vi "Sensor_Read_Val.vi"(10 "Ele_At_Pos":bool, 11 "Ref_Num":T23) -> (3 "Sensor_Val":T24)   [LabVIEW 2014]
uses:
  <vilib>/Rock Robotics/WPI/Joystick/WPI_JoystickDevRef.ctl
  <vilib>/Rock Robotics/WPI/Joystick/WPI_JoystickDeviceEnum.ctl
  <vilib>/Rock Robotics/WPI/RobotDrive/WPI_RobotDriveDevRef.ctl
  <vilib>/Rock Robotics/WPI/MotorControl/WPI_MotorControlDeviceRef.ctl
  <vilib>/Rock Robotics/WPI/MotorControl/WPI_MotorControlType.ctl
  <vilib>/Rock Robotics/SystemInterfaces/Typedef/FPGA_TypedefDigitalModule.ctl
  <vilib>/Rock Robotics/SystemInterfaces/DIO/FPGA_DIOPWMChannel.ctl
  <vilib>/Rock Robotics/WPI/PWM/WPI_PWMDeadband.ctl
  <vilib>/Rock Robotics/WPI/CAN/Jaguar/SubVIs/WPI_CANJaguar_ControlMode.ctl
  <vilib>/Rock Robotics/WPI/CAN/TalonSRX/WPI_CANTalonSRX_APIControlMode.ctl
  <vilib>/Rock Robotics/WPI/PWM/WPI_PWMTransform_ConPane.ctl
  <vilib>/Rock Robotics/WPI/Encoder/WPI_EncoderDevRef.ctl
  <vilib>/Rock Robotics/SystemInterfaces/Encoder/FPGA_EncoderIdx.ctl
  <vilib>/Rock Robotics/SystemInterfaces/Counter/FPGA_CounterCtrSystemIndex.ctl
  <vilib>/Rock Robotics/WPI/Encoder/WPI_EncoderType.ctl
  <vilib>/Rock Robotics/WPI/AnalogChannel/WPI_AnalogChannelDevRef.ctl
  <vilib>/Rock Robotics/SystemInterfaces/Typedef/FPGA_TypedefAnalogModule.ctl
  <vilib>/Rock Robotics/SystemInterfaces/AI/FPGA_AIChannel.ctl
  <vilib>/Rock Robotics/WPI/Gyro/WPI_GyroDevRef.ctl
  AdaIMU roboRIO/IMUDevRef.ctl
  <vilib>/Rock Robotics/SystemInterfaces/i2clib/i2c_bus.ctl
panel:
  in  "Reset Zero Position 2":bool
  in  "Detect_Tote_Thresh_Hold":dbl
  in  "Yoyo_Scale_to_Inch":dbl
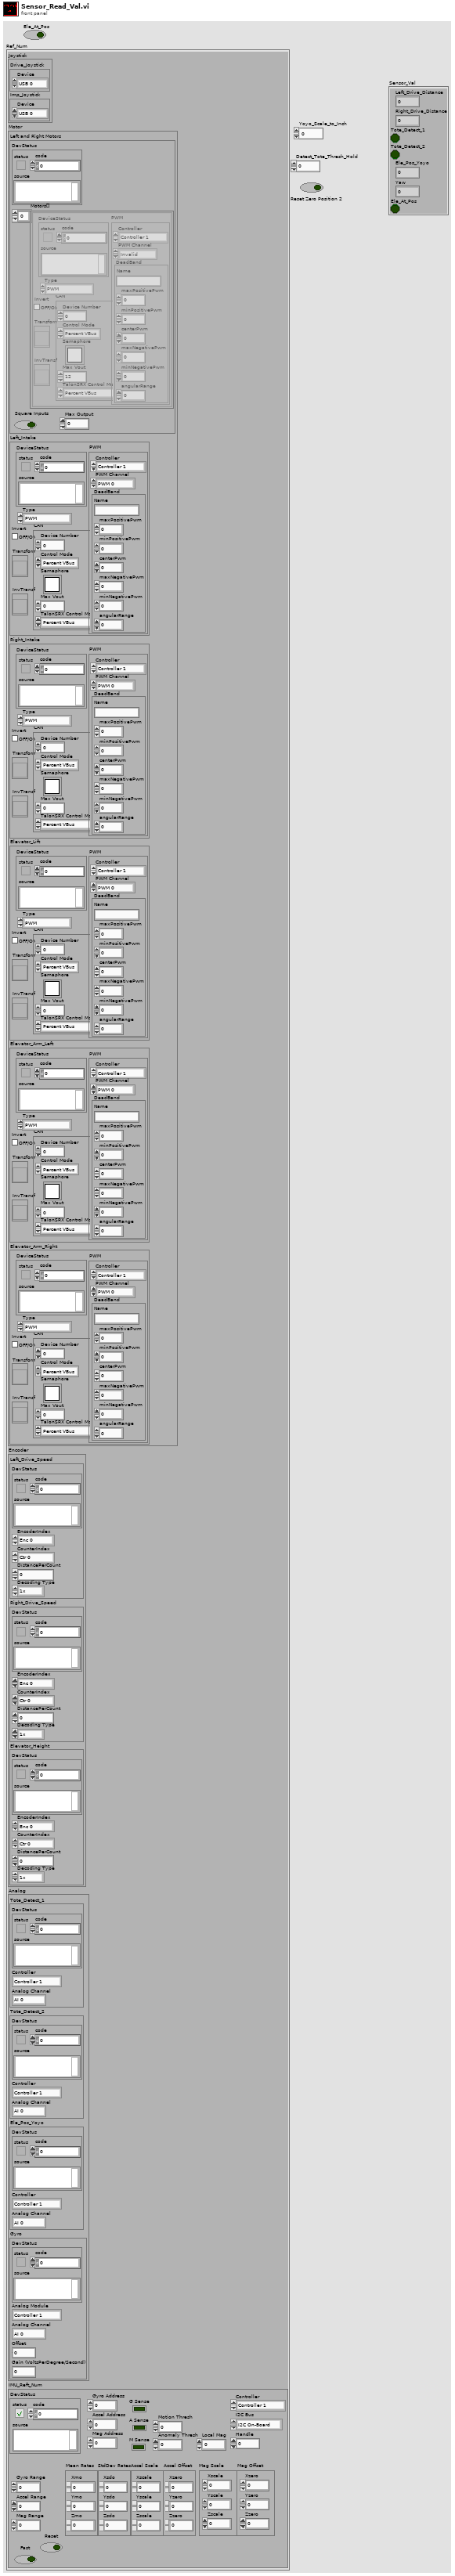
[diagram p1: front panel]
types:
  T1 = typedef "WPI_JoystickDevRef.ctl" = cluster{"Device":T2}
  T2 = typedef "WPI_JoystickDeviceEnum.ctl" = enum16{"USB 0", "USB 1", "USB 2", "USB 3", "USB 4", "USB 5"}
  T3 = typedef "WPI_RobotDriveDevRef.ctl" = cluster{"DevStatus":errorcluster, "Motors[]":T4[], "Square Inputs":bool, "Max Output":dbl}
  T4 = typedef "WPI_MotorControlDeviceRef.ctl" = cluster{"DeviceStatus":errorcluster, "Type":T5, "PWM":cluster{"Controller":T6, "PWM Channel":T7, "DeadBand":T8}, "CAN":cluster{"Device Number":u8, "Control Mode":T9, "Semaphore":T10, "Max Vout":dbl, "TalonSRX Control Mode":T11}, "Invert":bool, "TransformRef":T12, "InvTransformRef":T12}
  T5 = typedef "WPI_MotorControlType.ctl" = enum16{"PWM", "CAN", "CANTalonSRX"}
  T6 = typedef "FPGA_TypedefDigitalModule.ctl" = enum16{"Controller 1"}
  T7 = typedef "FPGA_DIOPWMChannel.ctl" = enum8{"PWM 0", "PWM 1", "PWM 2", "PWM 3", "PWM 4", "PWM 5", "PWM 6", "PWM 7", "PWM 8", "PWM 9", "PWM MXP 0", "PWM MXP 1", "PWM MXP 2", "PWM MXP 3", "PWM MXP 4", "PWM MXP 5", "PWM MXP 6", "PWM MXP 7", "PWM MXP 8", "PWM MXP 9", "Invalid"}
  T8 = typedef "WPI_PWMDeadband.ctl" = cluster{"Name":string, "maxPositivePwm":i32, "minPositivePwm":i32, "centerPwm":i32, "maxNegativePwm":i32, "minNegativePwm":i32, "angularRange":u16}
  T9 = typedef "WPI_CANJaguar_ControlMode.ctl" = enum8{"Percent VBus", "Current", "Speed", "Position", "Voltage"}
  T10 = typedef "Semaphore RefNum" = refnum<k1>
  T11 = typedef "WPI_CANTalonSRX_APIControlMode.ctl" = enum8{"Percent VBus", "Speed", "Position", "Slave", "Unchanged / Invalid"}
  T12 = typedef "WPI_PWMTransform_ConPane.ctl" = refnum<vi>
  T13 = typedef "WPI_EncoderDevRef.ctl" = cluster{"DevStatus":errorcluster, "EncoderIndex":T14, "CounterIndex":T15, "DistancePerCount":dbl, "Decoding Type":T16}
  T14 = typedef "FPGA_EncoderIdx.ctl" = enum8{"Enc 0", "Enc 1", "Enc 2", "Enc 3", "Enc 4", "Enc 5", "Enc 6", "Enc 7", "Invalid"}
  T15 = typedef "FPGA_CounterCtrSystemIndex.ctl" = enum8{"Ctr 0", "Ctr 1", "Ctr 2", "Ctr 3", "Ctr 4", "Ctr 5", "Ctr 6", "Ctr 7", "Invalid"}
  T16 = typedef "WPI_EncoderType.ctl" = enum16{"1x", "2x", "4x"}
  T17 = typedef "WPI_AnalogChannelDevRef.ctl" = cluster{"DevStatus":errorcluster, "Controller":T18, "Analog Channel":T19}
  T18 = typedef "FPGA_TypedefAnalogModule.ctl" = enum16{"Controller 1"}
  T19 = typedef "FPGA_AIChannel.ctl" = enum8{"AI 0", "AI 1", "AI 2", "AI 3", "AI MXP 0", "AI MXP 1", "AI MXP 2", "AI MXP 3", "Invalid"}
  T20 = typedef "WPI_GyroDevRef.ctl" = cluster{"DevStatus":errorcluster, "Analog Module":T18, "Analog Channel":T19, "Offset":dbl, "Gain (VoltsPerDegree/Second)":dbl}
  T21 = typedef "IMUDevRef.ctl" = cluster{"DevStatus":errorcluster, "Gyro Address":u8, "Gyro Range":u8, "Mean Rates":cluster{"Xmo":dbl, "Ymo":dbl, "Zmo":dbl}, "StdDev Rates":cluster{"Xsdo":dbl, "Ysdo":dbl, "Zsdo":dbl}, "Fast":bool, "Reset":bool, "Accel Address":u8, "Accel Range":u8, "Accel Scale":cluster{"Xscale":dbl, "Yscale":dbl, "Zscale":dbl}, "Mag Address":u8, "Mag Range":u8, "G Sense":bool, "A Sense":bool, "M Sense":bool, "Accel Offset":cluster{"Xzero":dbl, "Yzero":dbl, "Zzero":dbl}, "Motion Thresh":dbl, "Mag Scale":cluster{"Xscale":dbl, "Yscale":dbl, "Zscale":dbl}, "Mag Offset":cluster{"Xzero":dbl, "Yzero":dbl, "Zzero":dbl}, "I2C Bus":T22, "Handle":i32, "Controller":T6, "Anomaly Thresh":dbl, "Local Mag":dbl}
  T22 = typedef "i2c_bus.ctl" = enum16{"I2C On-Board", "I2C MXP", "Invalid"}
  T23 = cluster{"Joystick":cluster{"Drive_Joystick":T1, "Imp_Joystick":T1}, "Motor":cluster{"Left and Right Motors":T3, "Left_Intake":T4, "Right_Intake":T4, "Elevator_Lift":T4, "Elevator_Arm_Left":T4, "Elevator_Arm_Right":T4}, "Encoder":cluster{"Left_Drive_Speed":T13, "Right_Drive_Speed":T13, "Elevator_Height":T13}, "Analog":cluster{"Tote_Detect_1":T17, "Tote_Detect_2":T17, "Ele_Pos_Yoyo":T17, "Gyro":T20}, "IMU_Reft_Num":T21}
  T24 = cluster{"Left_Drive_Distance":dbl, "Right_Drive_Distance":dbl, "Tote_Detect_1":bool, "Tote_Detect_2":bool, "Ele_Pos_Yoyo":dbl, "Yaw":dbl, "Ele_At_Pos":bool}
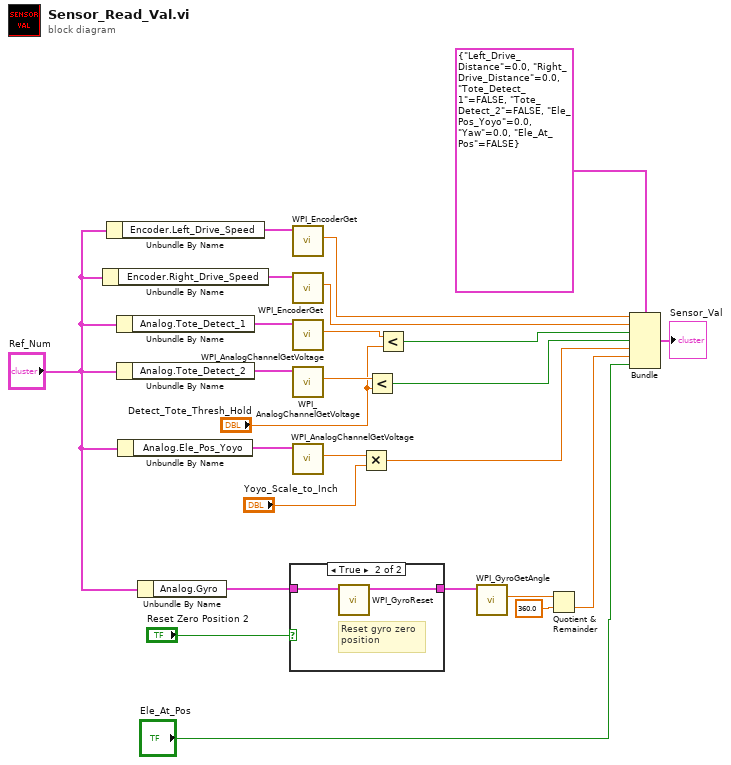
[diagram p0: block diagram]
diagram:
  n1 = Unbundle By Name("Ref_Num") -> ("Encoder.Right_Drive_Speed"=w15:T13)
  n2 = Unbundle By Name("Ref_Num") -> ("Encoder.Left_Drive_Speed"=w14:T13)
  n3 = Unbundle By Name("Ref_Num") -> ("Analog.Tote_Detect_1"=w16:T17)
  n4 = Unbundle By Name("Ref_Num") -> ("Analog.Tote_Detect_2"=w17:T17)
  n5 = Unbundle By Name("Ref_Num") -> ("Analog.Ele_Pos_Yoyo"=w18:T17)
  n6 = Unbundle By Name("Ref_Num") -> ("Analog.Gyro"=w22:T20)
  n7 = case shown="True" "Reset Zero Position 2" {
    tunnel: [w26 w28] -> w19
    tunnel: w22 -> [w26 w27]
    frame False {
    }
    frame True {
      # "Reset gyro zero \nposition"
      n8 = call <vilib>:"WPI_GyroReset.vi"("GyroDevRef"=w27) -> ("GyroDevRef"=w28:T20)  [unwired: 10 out]
    }
  }
  n9 = call <vilib>:"WPI_EncoderGet.vi"("EncoderDevRef"=w14) -> ("Distance"=w23:dbl)  [unwired: 5 in, 5 out]
  n10 = call <vilib>:"WPI_EncoderGet.vi"("EncoderDevRef"=w15) -> ("Distance"=w24:dbl)  [unwired: 5 in, 5 out]
  n11 = call <vilib>:"WPI_AnalogChannelGetVoltage.vi"("AIDeviceRef"=w16) -> ("Voltage"=w8:dbl)  [unwired: 8 in, 2 out]
  n12 = call <vilib>:"WPI_AnalogChannelGetVoltage.vi"("AIDeviceRef"=w17) -> ("Voltage"=w10:dbl)  [unwired: 8 in, 2 out]
  n13 = call <vilib>:"WPI_AnalogChannelGetVoltage.vi"("AIDeviceRef"=w18) -> ("Voltage"=w13:dbl)  [unwired: 8 in, 2 out]
  n14 = Multiply(x=w13, y="Yoyo_Scale_to_Inch") -> (x*y=w12:dbl)
  n15 = Less?(x=w10, y="Detect_Tote_Thresh_Hold") -> (x < y?=w9:bool)
  n16 = Less?(x=w8, y="Detect_Tote_Thresh_Hold") -> (x < y?=w6:bool)
  n17 = call <vilib>:"WPI_GyroGetAngle.vi"("GyroDevRef"=w19) -> ("Angle"=w20:dbl)  [unwired: 1 in, 9 out]
  n18 = Quotient & Remainder(x=w20, y=360.0) -> (floor(x/y)=w25:dbl)  [unwired: 1 out]
  n19 = Bundle(cluster=T24 {"Left_Drive_Distance"=0.0, "Right_Drive_Distance"=0.0, "Tote_Detect_1"=FALSE, "Tote_Detect_2"=FALSE, "Ele_Pos_Yoyo"=0.0, "Yaw"=0.0, "Ele_At_Pos"=FALSE}, "Left_Drive_Distance"=w23, "Right_Drive_Distance"=w24, "Tote_Detect_1"=w6, "Tote_Detect_2"=w9, "Ele_Pos_Yoyo"=w12, "Yaw"=w25, "Ele_At_Pos"="Ele_At_Pos") -> (→"Sensor_Val":T24)
